vi "Window-Coordinates List.vi"() -> ()   [LabVIEW 2013]
uses:
  User Interface/Windows/Coordinates list window/Typedefs/Coordinate list window refs.ctl
  User Interface/Windows/Coordinates list window/Globals/Coord window-Globals.vi
  <vilib>/Utility/cursorutil.llb/Set Cursor (Icon Pict).vi
panel:
  in  "Picture Map":picture
  out "Stage XYZ Position ind.":cluster{"X":sgl, "Y":sgl, "Z":sgl} caption="Stage Position" {"Z" format="Z:%#_g"; "Y" format="Y:%#_g"; "X" format="X:%#_g"}
  out "File name":string
  in  "Coord Listbox":i32[](listbox)
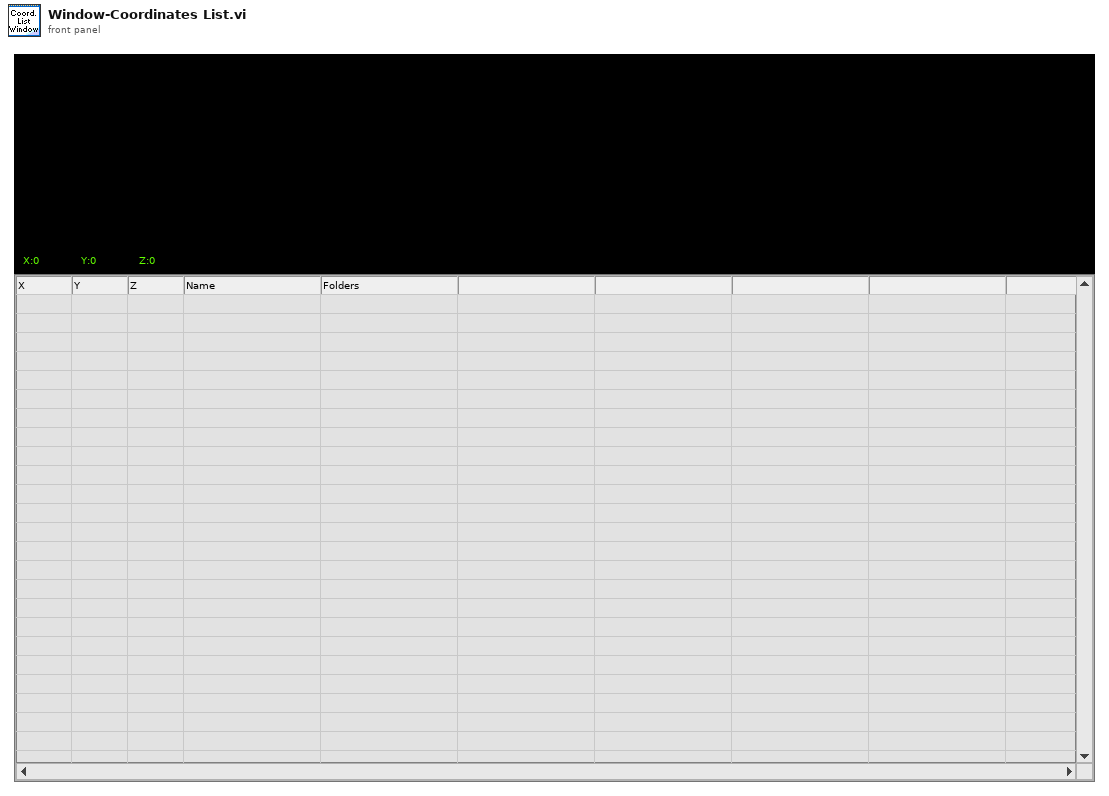
[diagram p1: front panel]
types:
  T1 = typedef "Coordinate list window refs.ctl" = cluster{"Window Name (i.e. Key)":string, "menu reference":refnum<k9>, "VI's reference":refnum<vi>, "Pane 1":refnum<vi>, "Pane 2":refnum<vi>, "Coord Listbox":refnum<vi>, "File name":refnum<vi>, "Picture Map":refnum<vi>, "Stage XYZ Position ind.":refnum<vi>}
  T2 = enum16{"Prevent horisontal resizing", "Prevent vertical resizing", "Prevent all resizing"}
  T3 = cluster{"Shift":bool, "Ctrl":bool, "Alt":bool, "Cmd":bool, "Opt":bool}
  T4 = typedef "eventvkey.ctl" = enum16{"ASCII", "Enter", "Return", "Shift", "Ctrl", "Alt", "Cmd", "Opt", "Caps", "NumLock", "Clear", "Break", "Up", "Down", "Left", "Right", "Insert", "Delete", "Home", "End", "PageUp", "PageDown", "Escape", "Help", "Pause", "ScrollLock", "F1", "F2", "F3", "F4", "F5", "F6", "F7", "F8", "F9", "F10", "F11", "F12", "F13", "F14", "F15", "F16", "F17", "F18", "F19", "F20", "F21", "F22", "F23", "F24", "Play", "VolumeUp", "VolumeDown", "Mute", "Two Byte Char"}
  T5 = typedef "LVPoint32TypeDef.ctl" = cluster{"Horizontal":i32, "Vertical":i32}
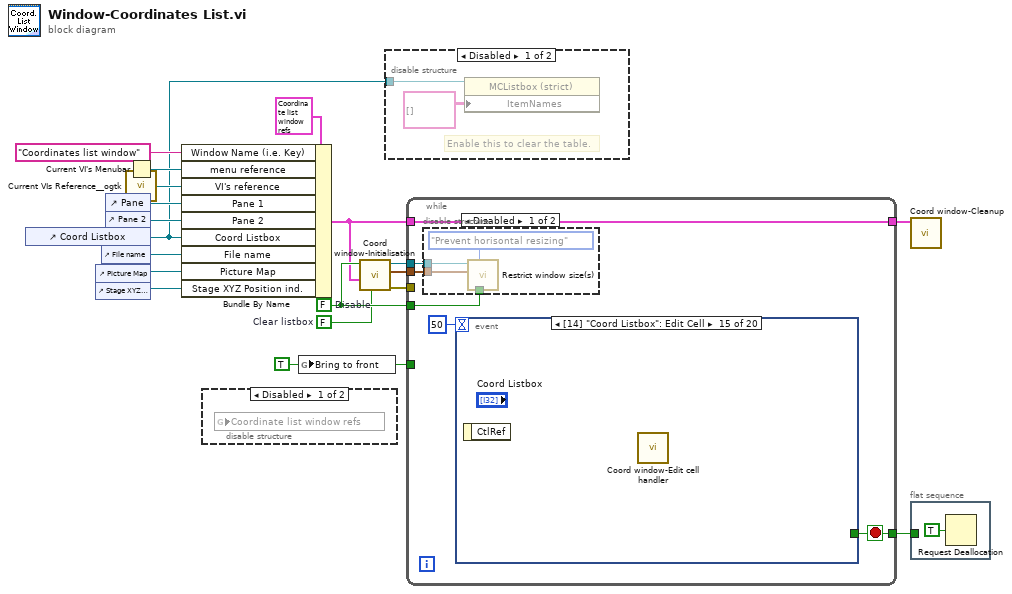
[diagram p0: block diagram]
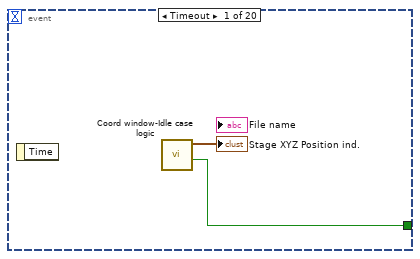
[diagram p5: hidden frame]
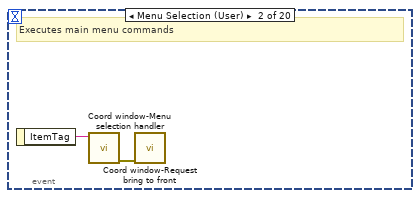
[diagram p6: hidden frame]
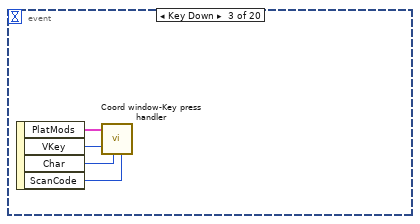
[diagram p7: hidden frame]
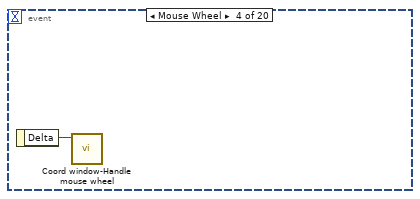
[diagram p8: hidden frame]
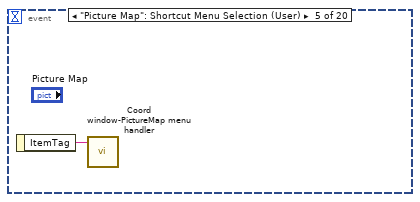
[diagram p9: hidden frame]
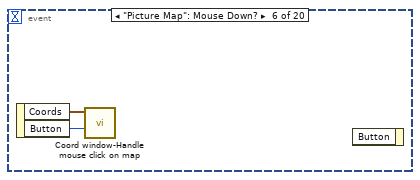
[diagram p10: hidden frame]
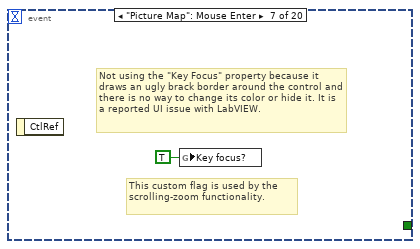
[diagram p11: hidden frame]
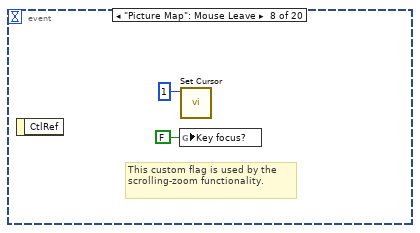
[diagram p12: hidden frame]
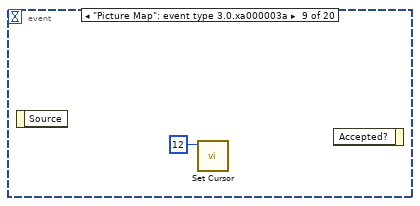
[diagram p13: hidden frame]
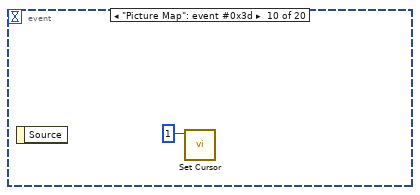
[diagram p14: hidden frame]
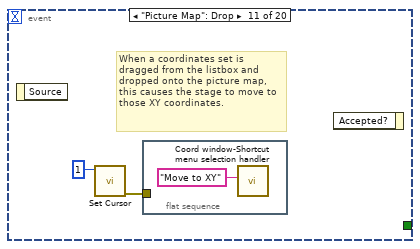
[diagram p15: hidden frame]
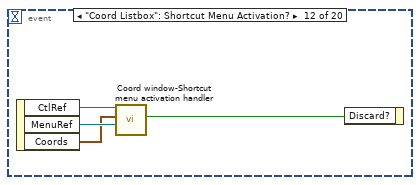
[diagram p16: hidden frame]
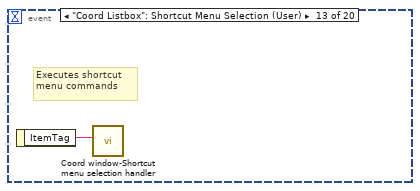
[diagram p17: hidden frame]
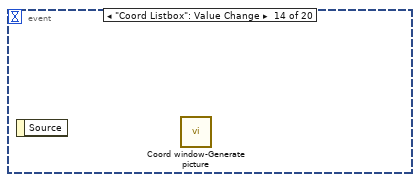
[diagram p18: hidden frame]
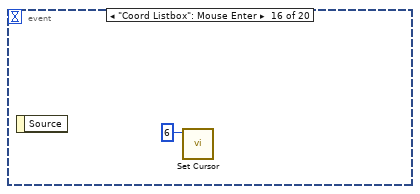
[diagram p19: hidden frame]
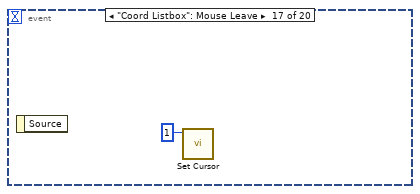
[diagram p20: hidden frame]
diagram:
  w1 = TRUE ("Bring to front")
  w5 = FALSE  # Clear listbox
  w9 = FALSE  # Disable
  n1 = control-ref of="Coord Listbox"() -> (w3:refnum<vi>)
  n2 = control-ref of="Picture Map"() -> (w16:refnum<vi>)
  n3 = control-ref of="Stage XYZ Position ind."() -> (w4:refnum<vi>)
  n4 = control-ref of="File name"() -> (w18:refnum<vi>)
  n5 = control-ref of="Pane"() -> (w13:refnum<vi>)
  n6 = control-ref of="Pane 2"() -> (w12:refnum<vi>)
  n7 = call "Current VIs Reference__ogtk.vi"() -> ("Current VI's reference"=w15:refnum<vi>)  [unwired: 5 in]
  n8 = Current VI's Menubar() -> (w14:refnum<k9>)
  n9 = Bundle By Name(cluster=T1 {"Window Name (i.e. Key)"="", "menu reference"=refnum, "VI's reference"=refnum, "Pane 1"=refnum, "Pane 2"=refnum, "Coord Listbox"=refnum, "File name"=refnum, "Picture Map"=refnum, "Stage XYZ Position ind."=refnum} ("Coordinate list window refs"), "Window Name (i.e. Key)"="Coordinates list window", "menu reference"=w14, "VI's reference"=w15, "Pane 1"=w13, "Pane 2"=w12, "Coord Listbox"=w3, "File name"=w18, "Picture Map"=w16, "Stage XYZ Position ind."=w4) -> (w6:T1)
  n10 = disable-structure shown="Disabled" {
    frame Disabled {
      n11 = global read "Coord window-Globals.vi" "Coordinate list window refs"() -> ()  [unwired: 1 in]
    }
    frame Enabled {
    }
  }
  n12 = global write "Coord window-Globals.vi" "Bring to front"(w1) -> ()
  n13 = call "Coord window-Initialisation.vi"("Force-clear Listbox"=w5, "Coordinate list window refs"=w6, "Disable window positioning"=w9) -> ("error out"=w11:errorcluster, "Window size"=w19:cluster{"Horisontal":i16, "Vertical":i16}, "VI out"=w8:refnum<vi>)  [unwired: 6 in]
  n14 = disable-structure shown="Disabled" {
    disable-tunnel: w3 -> [w20 _]
    frame Disabled {
      # "Enable this to clear the table."
      n15 = property class="MCListbox (strict)"(reference=w20, "ItemNames"=string[][] [] ("Item Names")) -> ()  [unwired: 1 in, 2 out]
    }
    frame Enabled {
    }
  }
  n16 = while {
    tunnel: w19 -> [w25]
    tunnel: w9 -> [w26]
    tunnel: w11 -> [_]
    tunnel: w8 -> [w24]
    tunnel: w6 -> [w23]
    tunnel: [w23] -> w7
    tunnel: [w22] -> w2
    tunnel: w1 -> [_]
    stop <- w22 stop-if-true
    n17 = disable-structure shown="Disabled" {
      disable-tunnel: w26 -> [w31 _]
      disable-tunnel: w25 -> [w29 _]
      disable-tunnel: w24 -> [w28 _]
      frame Disabled {
        n18 = call "Restrict window size(s).vi"("Disable in"=w31, "Function"=T2."Prevent horisontal resizing", "Window size"=w29, "VI in"=w28) -> ()  [unwired: 7 in, 1 out]
      }
      frame Enabled {
      }
    }
    n19 = event shown="[14] \"Coord Listbox\": Edit Cell" {
      selector: _ -> [_ _ _ _ _ _ _ _ _ _ _ _ _ _ _ _ _ _ _ _]
      dyn-events: _ -> [_ _ _ _ _ _ _ _ _ _ _ _ _ _ _ _ _ _ _ _]
      timeout: 50 -> [_ _ _ _ _ _ _ _ _ _ _ _ _ _ _ _ _ _ _ _]
      tunnel: [w32 _ _ _ _ _ _ _ _ _ _ _ _ _ _ _ _ _ _ TRUE] -> w22
      event Timeout {
        n20 = event-data() -> ()  [unwired: 1 in, 1 out]
        n21 = call "Coord window-Idle case logic.vi"() -> ("Stop application"=w32:bool, "Coordinates"=→"Stage XYZ Position ind.":cluster{"X":sgl, "Y":sgl, "Z":sgl})  [unwired: 10 in]
      }
      event Menu Selection (User) {
        # "Executes main menu commands"
        n22 = event-data() -> ("ItemTag"=w35:string)  [unwired: 1 in]
        n23 = call "Coord window-Menu selection handler.vi"("ItemTag"=w35) -> ("error out"=w34:errorcluster)  [unwired: 10 in]
        n24 = call "Coord window-Request bring to front.vi"("error in (no error)"=w34) -> ()  [unwired: 10 in, 1 out]
      }
      event Key Down {
        n25 = event-data() -> ("PlatMods"=w38:T3, "VKey"=w39:T4, "Char"=w37:i16, "ScanCode"=w36:i16)  [unwired: 1 in]
        n26 = call "Coord window-Key press handler.vi"("ScanCode"=w36, "Char"=w37, "VKey"=w39, "PlatMods"=w38) -> ()  [unwired: 8 in]
      }
      event Mouse Wheel {
        n27 = event-data() -> ("Delta"=w40:i32)  [unwired: 1 in]
        n28 = call "Coord window-Handle mouse wheel.vi"("Delta"=w40) -> ()  [unwired: 11 in]
      }
      event "Picture Map": Shortcut Menu Selection (User) {
        n29 = event-data() -> ("ItemTag"=w41:string)  [unwired: 1 in]
        n30 = call "Coord window-PictureMap menu handler.vi"("ItemTag"=w41) -> ()  [unwired: 11 in]
      }
      event "Picture Map": Mouse Down? {
        n31 = event-data() -> ("Coords"=w43:T5, "Button"=w42:u16)  [unwired: 1 in]
        n32 = call "Coord window-Handle mouse click on map.vi"("Button"=w42, "Coordinates of pixel clicked on"=w43) -> ()  [unwired: 10 in]
        n33 = event-data() -> ()  [unwired: 2 in, 1 out]
      }
      event "Picture Map": Mouse Enter {
        # "This custom flag is used by the scrolling-zoom functionality."
        # "Not using the \"Key Focus\" property because it draws an ugly brack border around the control and there is no way to change its color or hide it. It is a reported UI issue with LabVIEW."
        n34 = event-data() -> ()  [unwired: 1 in, 1 out]
        n35 = global write "Coord window-Globals.vi" "Key focus?"(TRUE ("Key Focus")) -> ()
      }
      event "Picture Map": Mouse Leave {
        # "This custom flag is used by the scrolling-zoom functionality."
        n36 = event-data() -> ()  [unwired: 1 in, 1 out]
        n37 = global write "Coord window-Globals.vi" "Key focus?"(FALSE ("Key Focus")) -> ()
        n38 = call-poly <vilib>:"Set Cursor.vi"("icon"=u16 1) -> ()  [unwired: 9 in, 2 out]
      }
      event "Picture Map": event type 3.0.xa000003a {
        n39 = event-data() -> ()  [unwired: 1 in, 1 out]
        n40 = call-poly <vilib>:"Set Cursor.vi"("icon"=u16 12) -> ()  [unwired: 9 in, 2 out]
        n41 = event-data() -> ()  [unwired: 2 in, 1 out]
      }
      event "Picture Map": event #0x3d {
        n42 = event-data() -> ()  [unwired: 1 in, 1 out]
        n43 = call-poly <vilib>:"Set Cursor.vi"("icon"=u16 1) -> ()  [unwired: 9 in, 2 out]
      }
      event "Picture Map": Drop {
        # "When a coordinates set is dragged from the listbox and dropped onto the picture map, this causes the stage to move to those XY coordinates."
        n44 = event-data() -> ()  [unwired: 1 in, 1 out]
        n45 = call-poly <vilib>:"Set Cursor.vi"("icon"=u16 1) -> ("error out"=w50:errorcluster)  [unwired: 9 in, 1 out]
        n46 = flat-sequence {
          tunnel: w50 -> [_]
          frame #0 {
            n47 = call "Coord window-Shortcut menu selection handler.vi"("Shortcut menu itemTag"="Move to XY") -> ()  [unwired: 10 in, 1 out]
          }
        }
        n48 = event-data() -> ()  [unwired: 2 in, 1 out]
      }
      event "Coord Listbox": Shortcut Menu Activation? {
        n49 = event-data() -> ("CtlRef"=w54:refnum<vi>, "MenuRef"=w55:refnum<k9>, "Coords"=w53:T5)  [unwired: 1 in]
        n50 = call "Coord window-Shortcut menu activation handler.vi"("MenuRef"=w55, "Coords"=w53, "MulticolumnListbox in"=w54) -> ("Clicked on empty row"=w52:bool)  [unwired: 5 in, 3 out]
        n51 = event-data("Discard?"=w52) -> ()  [unwired: 1 in, 1 out]
      }
      event "Coord Listbox": Shortcut Menu Selection (User) {
        # "Executes shortcut menu commands"
        n52 = event-data() -> ("ItemTag"=w56:string)  [unwired: 1 in]
        n53 = call "Coord window-Shortcut menu selection handler.vi"("Shortcut menu itemTag"=w56) -> ()  [unwired: 10 in, 1 out]
      }
      event "Coord Listbox": Value Change {
        n54 = event-data() -> ()  [unwired: 1 in, 1 out]
        n55 = call "Coord window-Generate picture.vi"() -> ()  [unwired: 11 in, 1 out]
      }
      event "Coord Listbox": Edit Cell {
        n56 = event-data() -> ()  [unwired: 1 in, 1 out]
        n57 = call "Coord window-Edit cell handler.vi"() -> ()  [unwired: 12 in]
      }
      event "Coord Listbox": Mouse Enter {
        n58 = event-data() -> ()  [unwired: 1 in, 1 out]
        n59 = call-poly <vilib>:"Set Cursor.vi"("icon"=u16 6) -> ()  [unwired: 9 in, 2 out]
      }
      event "Coord Listbox": Mouse Leave {
        n60 = event-data() -> ()  [unwired: 1 in, 1 out]
        n61 = call-poly <vilib>:"Set Cursor.vi"("icon"=u16 1) -> ()  [unwired: 9 in, 2 out]
      }
      event "Coord Listbox": Drag Starting {
        n62 = event-data() -> ()  [unwired: 1 in, 1 out]
        n63 = call-poly <vilib>:"Set Cursor.vi"("icon"=u16 1) -> ()  [unwired: 9 in, 2 out]
      }
      event "Coord Listbox": Drag Ended {
        n64 = event-data() -> ()  [unwired: 1 in, 1 out]
        n65 = call-poly <vilib>:"Set Cursor.vi"("icon"=u16 6) -> ()  [unwired: 9 in, 2 out]
      }
      event Panel Close? {
        n66 = event-data() -> ()  [unwired: 1 in, 1 out]
        n67 = call "Coord window-Panel close handler.vi"() -> ()  [unwired: 12 in]
        n68 = event-data("Discard?"=FALSE) -> ()  [unwired: 1 in, 1 out]
      }
    }
  }
  n69 = call "Coord window-Cleanup.vi"("Coordinate list window refs"=w7) -> ()  [unwired: 11 in]
  n70 = flat-sequence {
    tunnel: w2 -> [_]
    frame #0 {
      n71 = Request Deallocation(TRUE ("flag")) -> ()
    }
  }
